vi "to string.vi"(8 "error in":errorcluster, 11 "CVT configuration in":refnum<class "testmod configuration.lvclass">) -> (0 "error out":errorcluster, 1 "data":string, 2 "version":string, 3 "CVT configuration out":refnum<class "testmod configuration.lvclass">)   [LabVIEW 2013, in "testmod configuration.lvclass"]
doc: "Provides an interface for saving a module configuration to a file or other serialized data source. It is recommended that all children of this class store data in two sets--data required for its own initialization, and any data required for parent initialization--and that each implementation uses the <b>Call Parent Method</b> primitive to serialize parent information."
uses:
  testmod configuration.lvclass
  <vilib>/NI/Tag Bus Module Framework/module configuration/TBM module configuration.lvclass
  testmod configuration.lvclass/testmod configuration.ctl
  <vilib>/NI/Tag Bus Module Framework/root configuration/unwrap data.vi
  <vilib>/NI/Tag Bus Module Framework/root configuration/TBM configuration.lvclass
  <vilib>/NI/CEF/CEF_TreeControl/serializable configuration/NISE_CEF_serializable configuration.lvclass
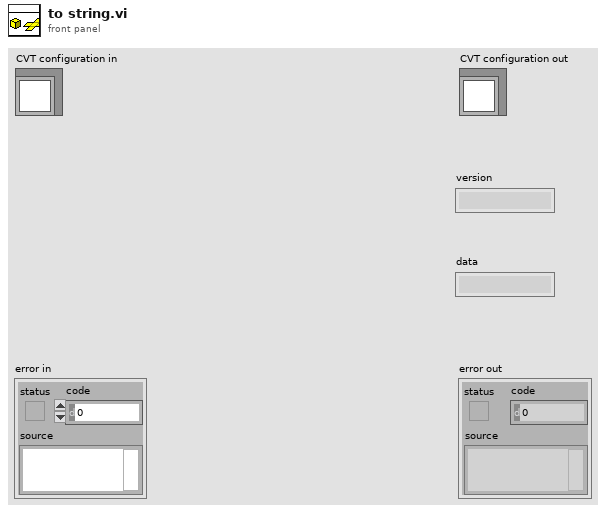
[diagram p1: front panel]
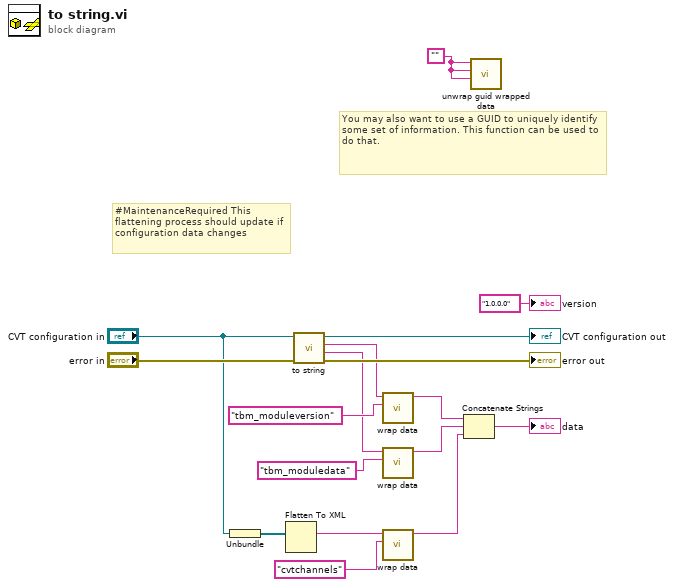
[diagram p0: block diagram]
diagram:
  w8 = ""
  # "You may also want to use a GUID to uniquely identify some set of information. This function can be used to do that."
  # "#MaintenanceRequired This flattening process should update if configuration data changes"
  n1 = Unbundle("CVT configuration in") -> (w5:refnum<class "TBM channel.lvclass">[])
  n2 = Flatten To XML(anything=w5) -> (xml string=w4:string)
  n3 = call-parent "to string.vi"("error in"="error in", "module configuration in"="CVT configuration in") -> ("error out"=→"error out":errorcluster, "data"=w9:string, "version"=w10:string, "module configuration out"=→"CVT configuration out":refnum<class "testmod configuration.lvclass">)  [unwired: 6 in]
  n4 = call <vilib>:"wrap data.vi"("identifier"="tbm_moduleversion" ("additional identifier"), "data to wrap"=w10) -> ("wrapped data"=w12:string)  [unwired: 9 in]
  n5 = call <vilib>:"wrap data.vi"("identifier"="tbm_moduledata" ("additional identifier"), "data to wrap"=w9) -> ("wrapped data"=w11:string)  [unwired: 9 in]
  n6 = call <vilib>:"wrap data.vi"("identifier"="cvtchannels" ("additional identifier"), "data to wrap"=w4) -> ("wrapped data"=w3:string)  [unwired: 9 in]
  n7 = Concatenate Strings(w12, w11, w3) -> (→"data":string)
  n8 = call <vilib>:"unwrap guid wrapped data.vi"("identifier"=w8, "uuid"=w8, "data to unwrap"=w8) -> ()  [unwired: 7 in, 2 out]
  "version" <- "1.0.0.0" ("version")
